vi "HacerFlipFlopJK.vi"() -> ()   [LabVIEW 2018]
panel:
  in  "K":bool=TRUE
  in  "J":bool=TRUE
  out "Q*":bool
  in  "stop":bool
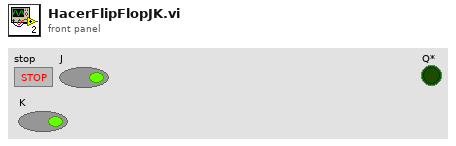
[diagram p1: front panel]
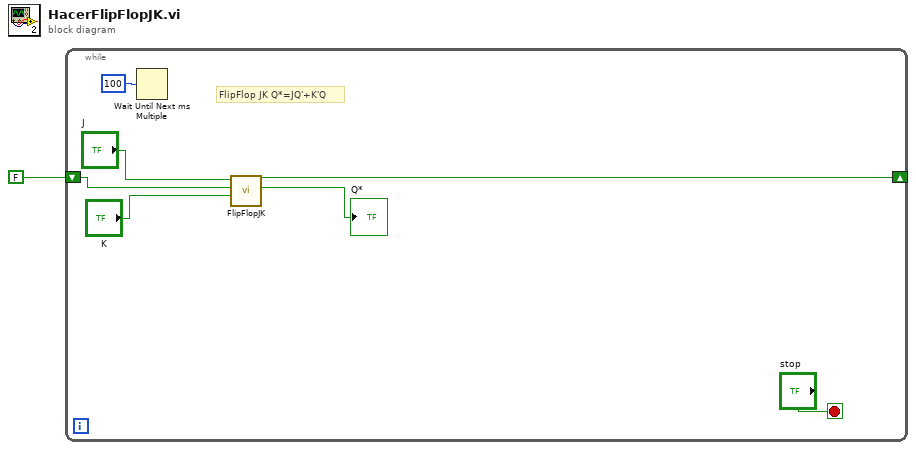
[diagram p0: block diagram]
diagram:
  n1 = while {
    shift-right: [w6] -> _
    shift-left: FALSE -> [w3]
    stop <- "stop" stop-if-true
    # "FlipFlop JK Q*=JQ'+K'Q"
    n2 = Wait Until Next ms Multiple(millisecond multiple=u32 100) -> ()  [unwired: 1 out]
    n3 = call "FlipFlopJK.vi"("K"="K", "Boolean in"=w3, "J"="J") -> ("Q*"=→"Q*":bool, "Boolean out"=w6:bool)  [unwired: 7 in]
  }
